vi "计算反射系数r.vi"(8 "x3":dbl, 9 "x1":dbl, 10 "H13":cdb[](array[numeric]), 11 "k":cdb[](array[numeric])) -> (3 "r complex":cdb[](array[numeric]))   [LabVIEW 2018]
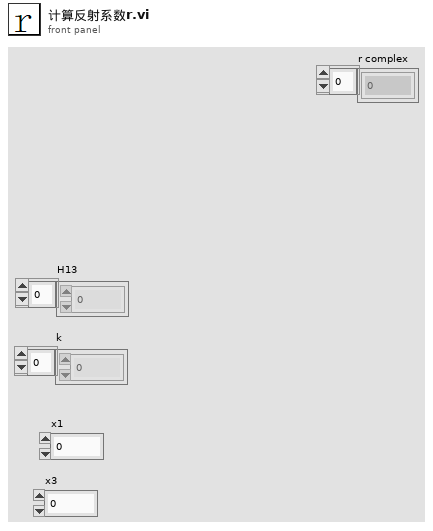
[diagram p1: front panel]
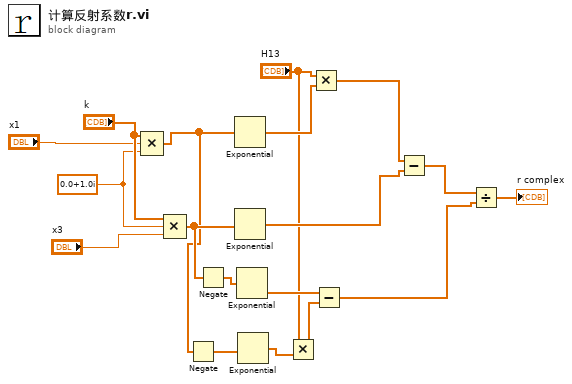
[diagram p0: block diagram]
diagram:
  w15 = cdb 0.0+1.0i ("数值")
  n1 = Compound Arithmetic op=MULTIPLY("k", "x1", w15) -> (w1:cdb[])
  n2 = Compound Arithmetic op=MULTIPLY("k", w15, "x3") -> (w11:cdb[])
  n3 = Negate(x=w1) -> (-x=w7:cdb[])
  n4 = Negate(x=w11) -> (-x=w10:cdb[])
  n5 = Exponential(1:w1) -> (0:w18:cdb[])
  n6 = Exponential(1:w11) -> (0:w12:cdb[])
  n7 = Exponential(1:w10) -> (0:w9:cdb[])
  n8 = Exponential(1:w7) -> (0:w6:cdb[])
  n9 = Multiply(x="H13", y=w6) -> (x*y=w5:cdb[])
  n10 = Multiply(x="H13", y=w18) -> (x*y=w17:cdb[])
  n11 = Subtract(x=w9, y=w5) -> (x-y=w4:cdb[])
  n12 = Subtract(x=w17, y=w12) -> (x-y=w13:cdb[])
  n13 = Divide(x=w13, y=w4) -> (x/y=→"r complex":cdb[])
